vi "Query Crest Factor.vi"(8 "error in (no error)":errorcluster, 11 "VISA resource name":refnum<visa-resource-name>) -> (0 "error out":errorcluster, 2 "Crest Factor":i32, 3 "VISA resource name out":refnum<visa-resource-name>)   [LabVIEW 2016, in "Yokogawa WT300 Series.lvlib"]
doc: "Queries the instrument crest factor."
uses:
  Yokogawa WT300 Series.lvlib
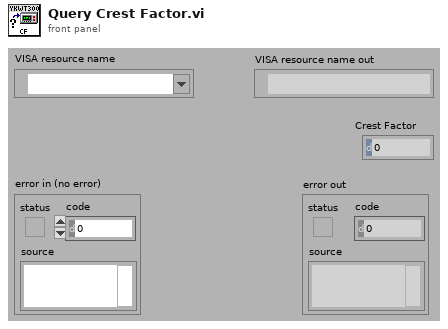
[diagram p1: front panel]
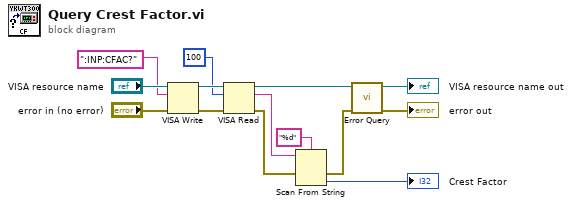
[diagram p0: block diagram]
diagram:
  n1 = VISA Write ("VISA書き込み")(VISA resource name="VISA resource name", write buffer=":INP:CFAC?", error in (no error)="error in (no error)") -> (VISA resource name out=w13:refnum<visa-resource-name>, error out=w14:errorcluster)  [unwired: 1 out]
  n2 = VISA Read ("VISA読み取り")(VISA resource name=w13, byte count=u32 100, error in (no error)=w14) -> (VISA resource name out=w5:refnum<visa-resource-name>, read buffer=w8:string, error out=w6:errorcluster)  [unwired: 1 out]
  n3 = Scan From String ("文字列からスキャン")(format string="%d", input string=w8, error in=w6) -> (error out=w3:errorcluster, output 1=→"Crest Factor":i32)  [unwired: 2 in, 2 out]
  n4 = call "Error Query.vi"("error in (no error)"=w3, "VISA resource name"=w5) -> ("error out"=→"error out":errorcluster, "VISA resource name out"=→"VISA resource name out":refnum<visa-resource-name>)  [unwired: 6 in, 2 out]
